vi "cmc_Pressure_Sensor.vi"() -> ()   [LabVIEW 2010]
panel:
  out "Low Pressure":bool[](array[boolean])
  out "High Pressure":bool[](array[boolean])
  in  "Delay Time (s)":dbl=1.0
  out "Waveform Chart":waveform(dbl)(graph)
  in  "stop":bool
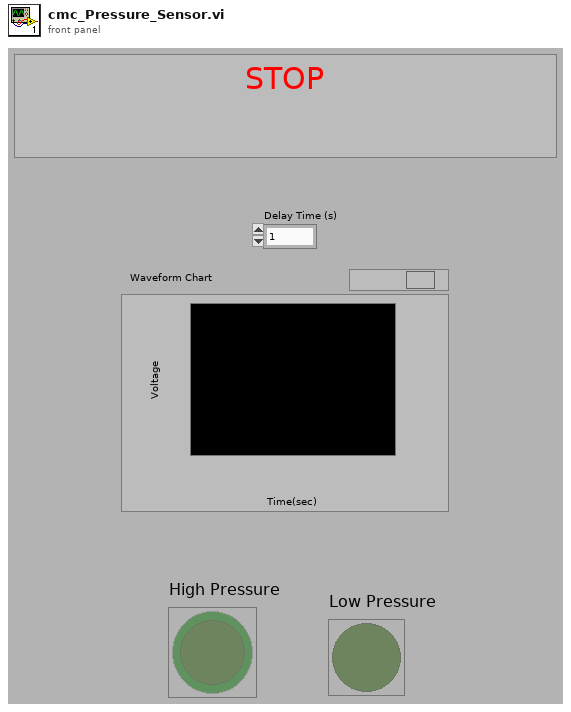
[diagram p1: front panel]
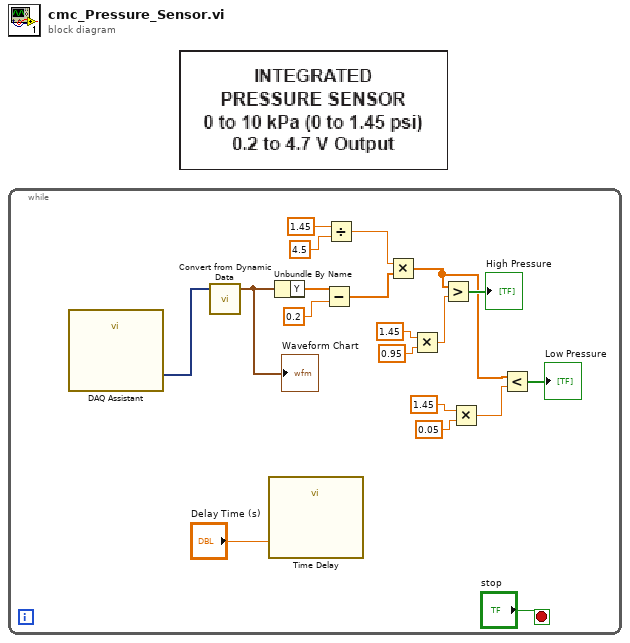
[diagram p0: block diagram]
diagram:
  n1 = while {
    stop <- "stop" stop-if-true
    n2 = call "DAQ Assistant"() -> ("data"=w17:dynamicdata)  [unwired: 17 in, 2 out]
    n3 = call "Convert from Dynamic Data"("Dynamic Data Type"=w17) -> ("Waveform"=w16:waveform(dbl))  [unwired: 3 in]
    "Waveform Chart" <- w16
    n4 = call "Time Delay"("Delay Time (s)"="Delay Time (s)") -> ()  [unwired: 10 in, 1 out]
    n5 = Unbundle By Name(w16) -> ("Y"=w15:dbl[])
    n6 = Subtract(x=w15, y=0.2) -> (x-y=w10:dbl[])
    n7 = Divide(x=1.45, y=4.5) -> (x/y=w11:dbl)
    n8 = Multiply(x=w11, y=w10) -> (x*y=w3:dbl[])
    n9 = Multiply(x=1.45, y=0.95) -> (x*y=w5:dbl)
    n10 = Greater?(x=w3, y=w5) -> (0:→"High Pressure":bool[])
    n11 = Multiply(x=1.45, y=0.05) -> (x*y=w2:dbl)
    n12 = Less?(x=w3, y=w2) -> (x < y?=→"Low Pressure":bool[])
  }
